vi "My Controls Example With MathScript VI.vi"() -> ()   [LabVIEW 2016]
uses:
  <vilib>/imath/engines/lvmath/Plug In/Control Design/BuiltInFunctions/tf/NIMS_CD_tf(num,den,Ts).vi
  <vilib>/imath/engines/lvmath/Plug In/Control Design/BuiltInFunctions/step/NIMS_CD_[Y,T]=step(TF,[Tinfo]).vi
  <vilib>/imath/engines/lvmath2/RunTimeEngine/NodeEndStatement/NIMS_NodeEndStatement_Get Vector.vi
  <instcachedir>/0/NIMS_NodeEndStatement_Get Vector_9E4547DF38A84F62A7E036B4CE3D251C.lvgen/NIMS_NodeEndStatement_Get Vector_9E4547DF38A84F62A7E036B4CE3D251C_001.vi
  <vilib>/imath/engines/lvmath2/RunTimeEngine/NodeEndStatement/NIMS_NodeEndStatement_Output.vi
  <instcachedir>/0/NIMS_NodeEndStatement_Output_53EC0D466D134D7ABD903AC30B43404B.lvgen/NIMS_NodeEndStatement_Output_53EC0D466D134D7ABD903AC30B43404B_005.vi
  <vilib>/imath/engines/lvmath2/RunTimeEngine/ErrorHandling/NIMS_Finalize Error.vi
panel:
  out "Step Response":dbl[](graph)
  in  "stop":bool
  in  "Natural Frequency":dbl(slide) scale=0.0..5.0
  in  "Damping Ratio":dbl(slide) scale=0.0..1.0
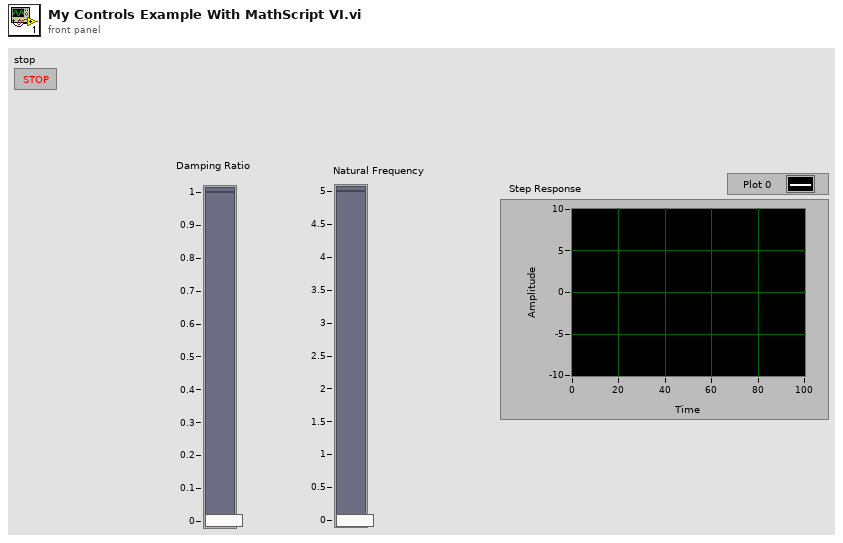
[diagram p1: front panel]
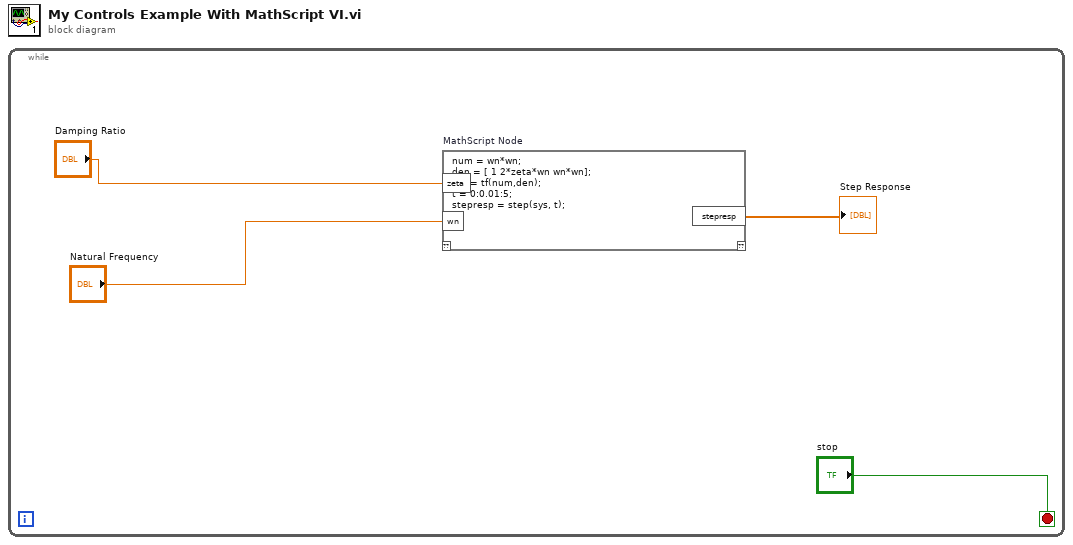
[diagram p0: block diagram]
diagram:
  n1 = while {
    stop <- "stop" stop-if-true
    n2 = mathscript code="num = wn*wn;\nden = [ 1 2*zeta*wn wn*wn];\nsys = tf(num,den);\nt = 0:0.01:5;\nstepresp = step(sys, t);"("zeta"="Damping Ratio", "wn"="Natural Frequency") -> ("stepresp"=→"Step Response":dbl[])  [unwired: 1 in, 1 out]
  }
